vi "Traction Receipe Trial.vi"() -> ()   [LabVIEW 2025]
panel:
  out "sum":dbl
  in  "SRR Sweep Range (%) 2":string caption="Speed (mm/s)"
  in  "Multicolumn Listbox":i32(listbox)
  in  "Total Execution Time":dbl
  in  "Total Steps":dbl
  in  "Duration / Step (s)":dbl=6.0
  in  "STRIBECK Fixed SRR List (%)":string="5,10,20,40,60,80,100"
  in  "Duration / Step (s)":dbl=6.0
  in  "SRR Sweep Range (%)":string
  in  "Rolling Speed (mm/s)":dbl=1000.0
  in  "Temperature Stages (°C)":string="40,100,140"
  in  "Ball Load (N)":string="25"
  in  "Lubricant Name":string
  in  "Profile File Name":string
  # "1. Test Identification & Global Setup"
  # "2. Step Configurations & Timing"
  # "Step 1 Configuration: TRACTION Step"
  # "%"
  # "Steps 2+ Configuration: STRIBECK Steps"
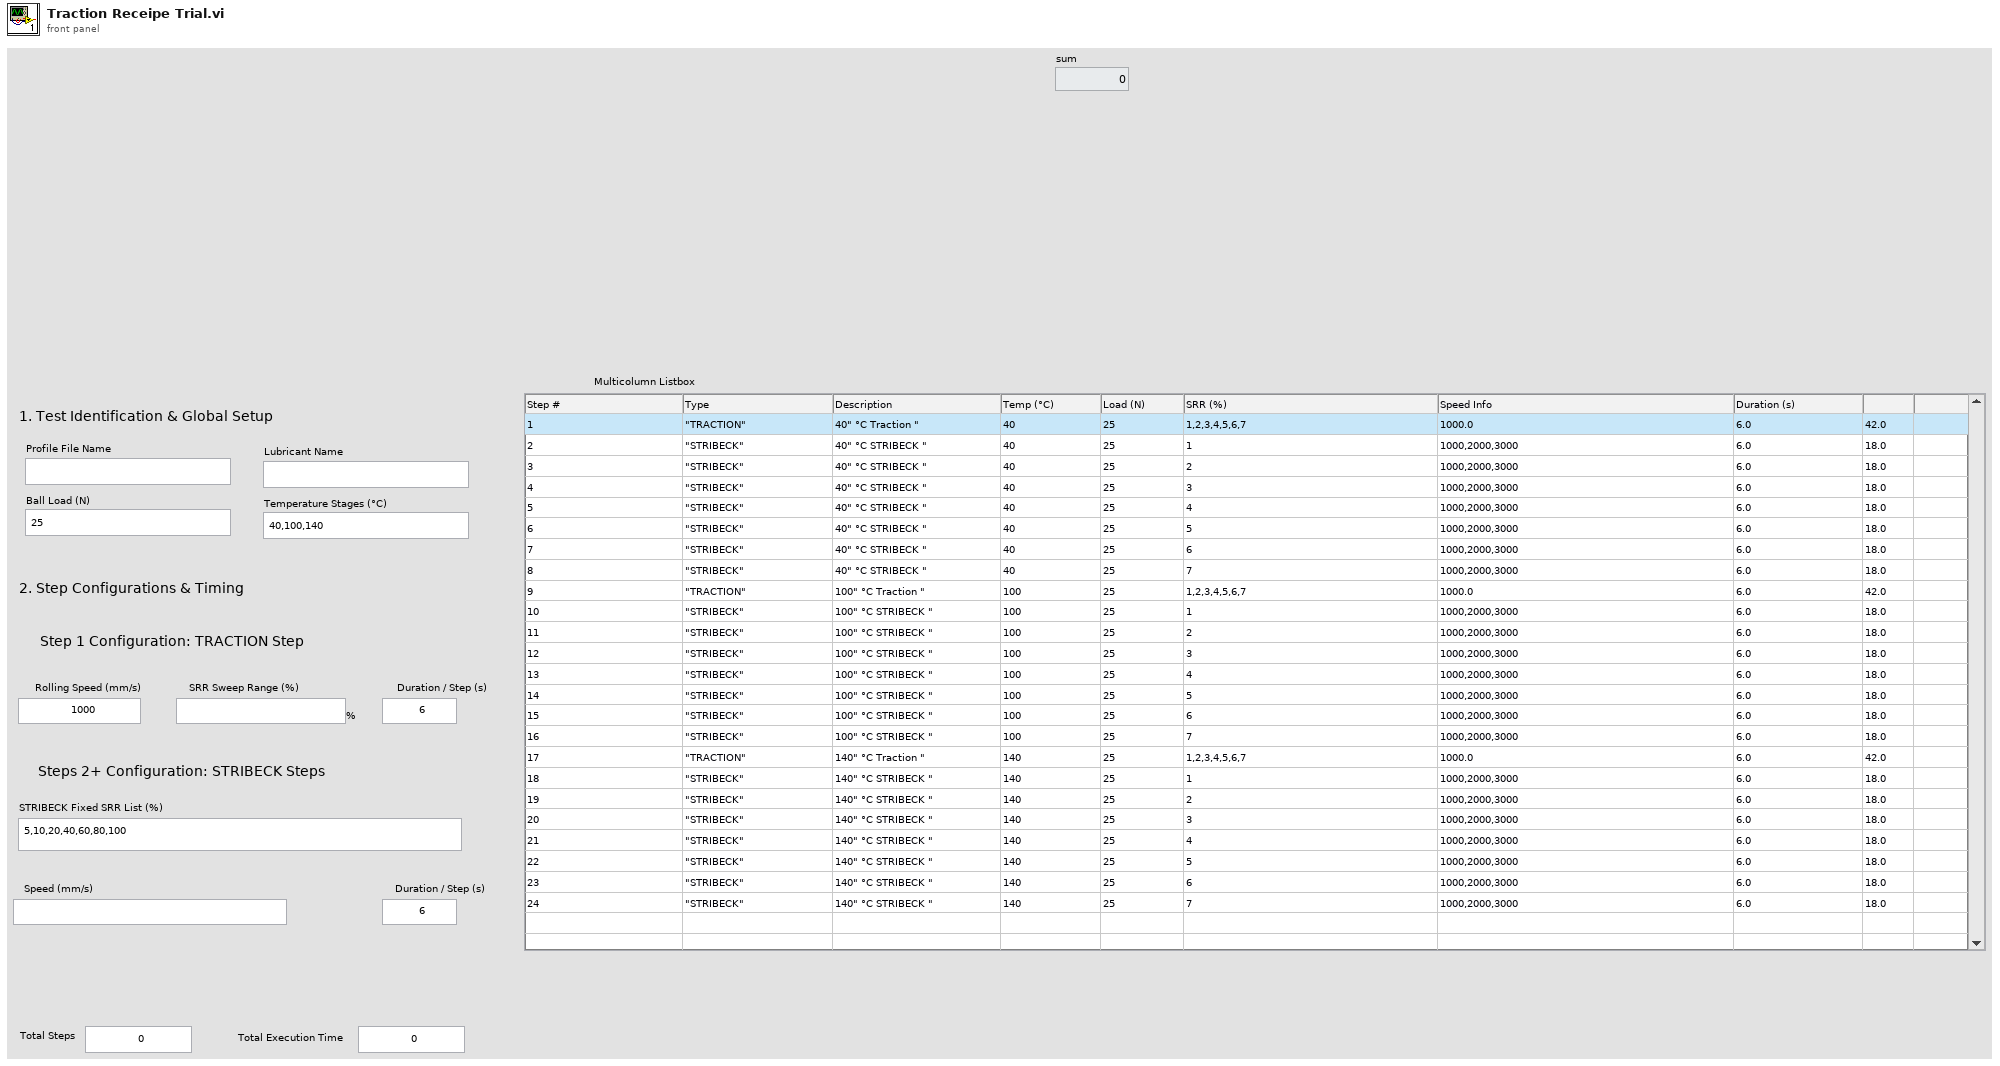
[diagram p1: front panel]
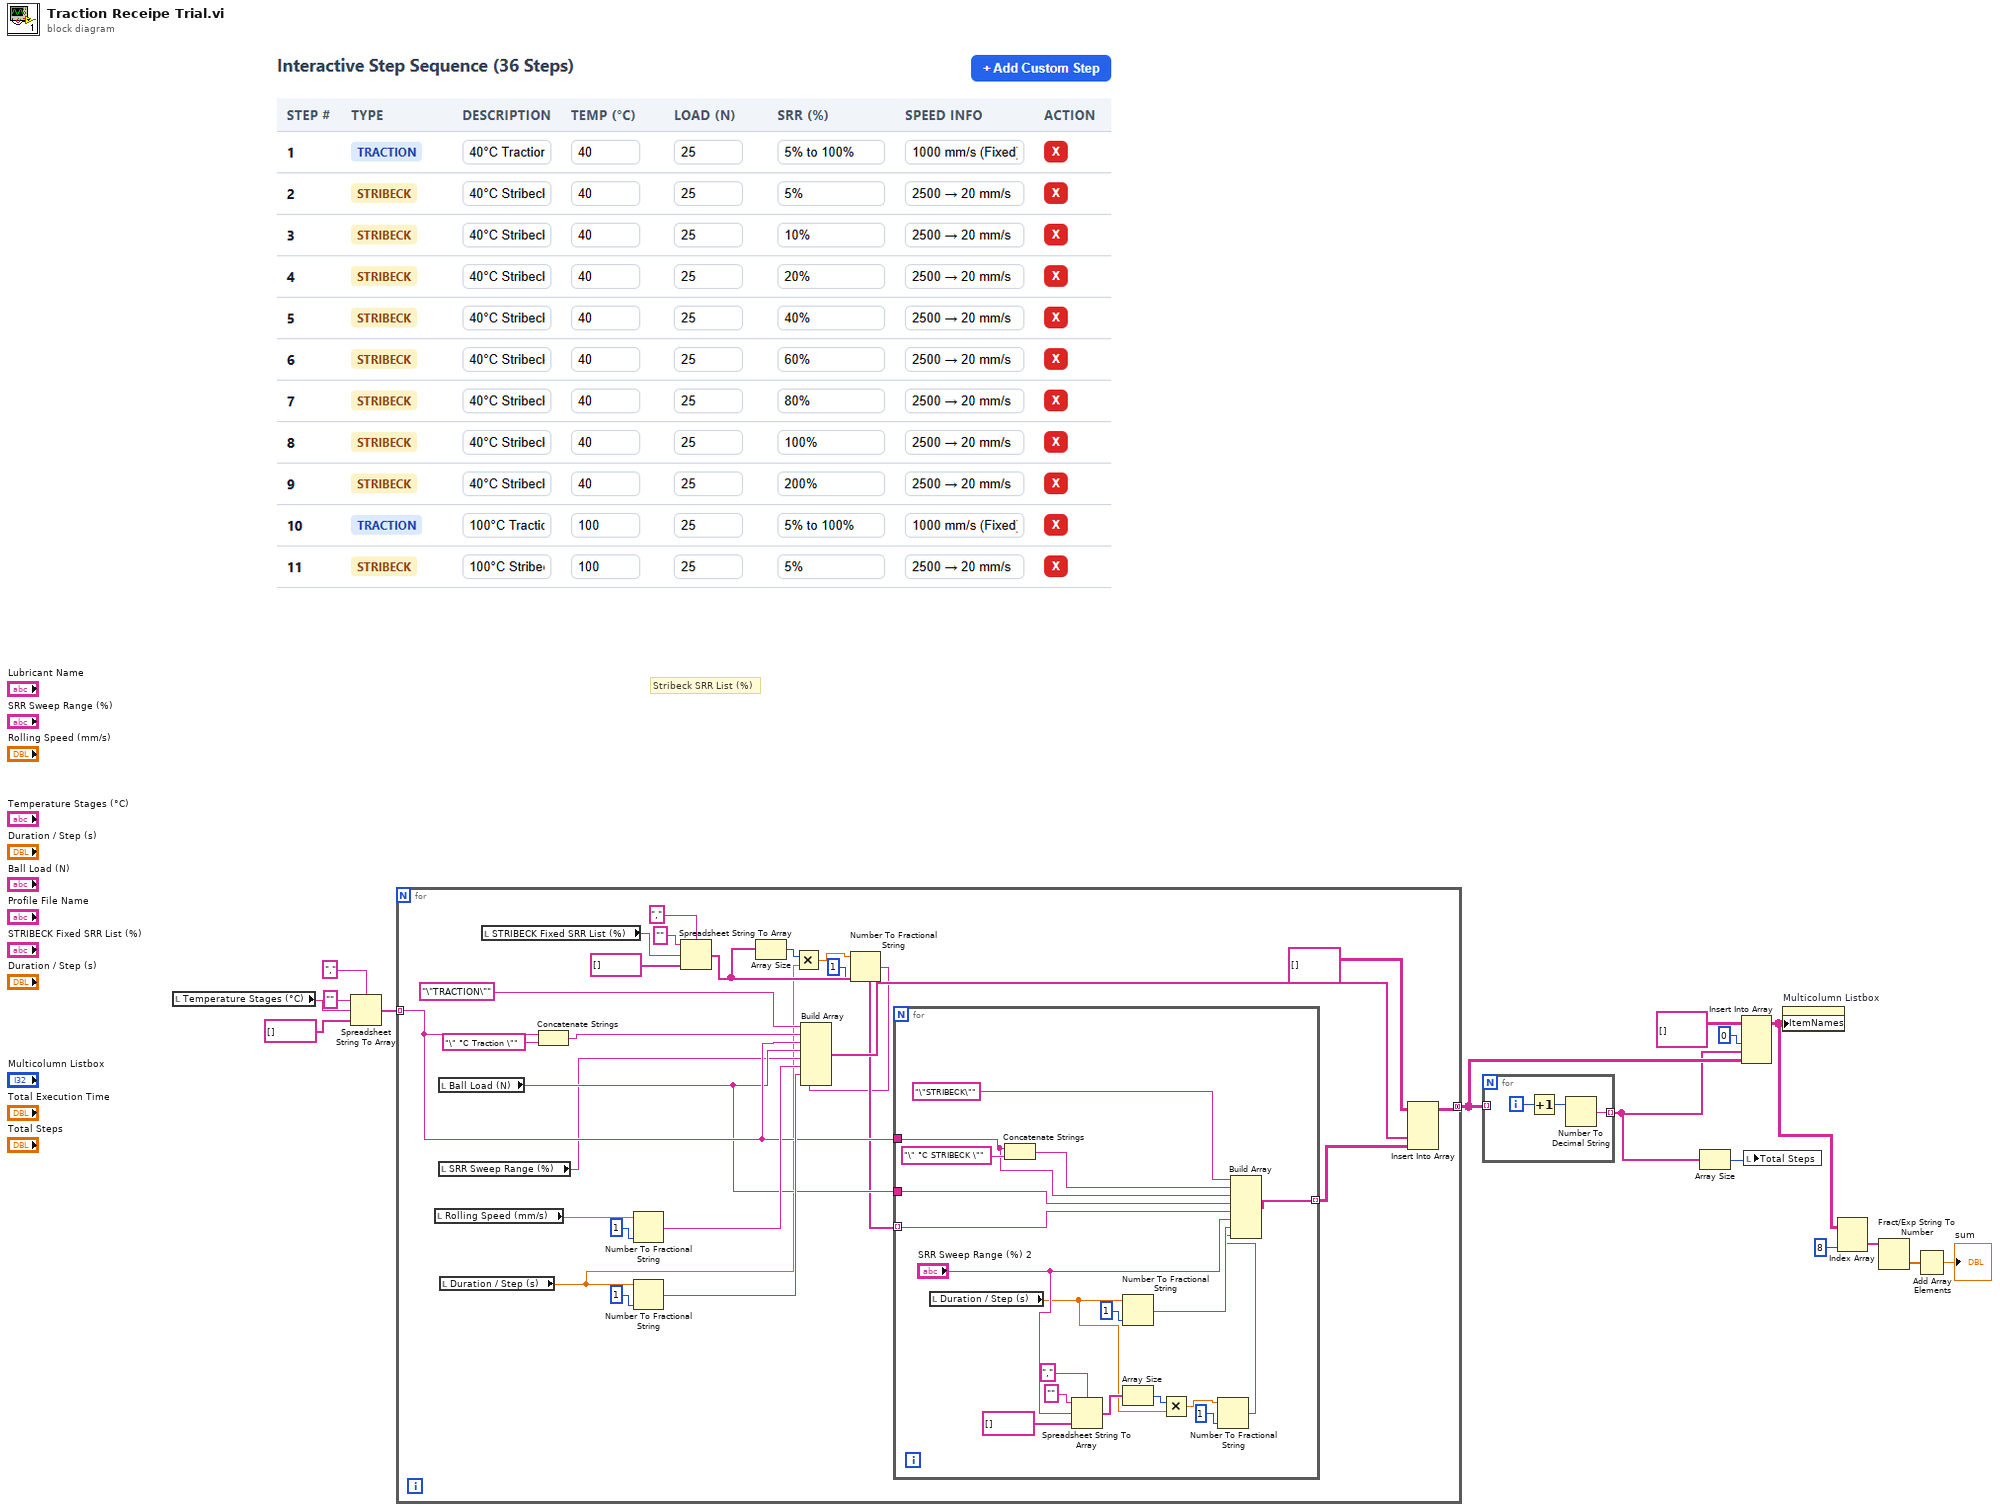
[diagram p0: block diagram]
diagram:
  # "Stribeck SRR List (%)"
  n1 = local read "Temperature Stages (°C)"() -> (w15:string)
  n2 = Spreadsheet String To Array(delimiter (Tab)=",", format string="", spreadsheet string=w15, array type (2D Dbl)=string[] []) -> (array=w11:string[])
  n3 = for {
    tunnel: w11 -> [w28] mode=indexing
    tunnel: [w23] -> w8 mode=concatenating
    n4 = local read "Rolling Speed (mm/s)"() -> (w38:dbl)
    n5 = local read "Ball Load (N)"() -> (w27:string)
    n6 = local read "SRR Sweep Range (%)"() -> (w22:string)
    n7 = local read "Duration / Step (s)"() -> (w19:dbl)
    n8 = local read "STRIBECK Fixed SRR List (%)"() -> (w32:string)
    n9 = Concatenate Strings(w28, "\" °C Traction \"" ("string")) -> (w35:string)
    n10 = Number To Fractional String(number=w38, precision (6)=i16 1) -> (F-format string=w34:string)  [unwired: 2 in]
    n11 = Number To Fractional String(number=w19, precision (6)=i16 1) -> (F-format string=w33:string)  [unwired: 2 in]
    n12 = Spreadsheet String To Array(delimiter (Tab)=",", format string="", spreadsheet string=w32, array type (2D Dbl)=string[] []) -> (array=w21:string[])
    n13 = Array Size(array=w21) -> (size(s)=w20:i32)
    n14 = Multiply(x=w20, y=w19) -> (x*y=w17:dbl)
    n15 = Number To Fractional String(number=w17, precision (6)=i16 1) -> (F-format string=w16:string)  [unwired: 2 in]
    n16 = Build Array("\"TRACTION\"", w35, w28, w27, w22, w34, w33, w16) -> (w25:string[])
    n17 = for {
      tunnel: w21 -> [w53] mode=indexing
      tunnel: w28 -> [w55]
      tunnel: w27 -> [w54]
      tunnel: [w51] -> w24 mode=indexing
      n18 = local read "Duration / Step (s)"() -> (w42:dbl)
      n19 = Concatenate Strings(w55, "\" °C STRIBECK \"" ("string")) -> (w56:string)
      n20 = Spreadsheet String To Array(delimiter (Tab)=",", format string="", spreadsheet string="SRR Sweep Range (%) 2", array type (2D Dbl)=string[] []) -> (array=w43:string[])
      n21 = Number To Fractional String(number=w42, precision (6)=i16 1) -> (F-format string=w52:string)  [unwired: 2 in]
      n22 = Array Size(array=w43) -> (size(s)=w46:i32)
      n23 = Multiply(x=w46, y=w42) -> (x*y=w44:dbl)
      n24 = Number To Fractional String(number=w44, precision (6)=i16 1) -> (F-format string=w41:string)  [unwired: 2 in]
      n25 = Build Array("\"STRIBECK\"", w56, w55, w54, w53, "SRR Sweep Range (%) 2", w52, w41) -> (w51:string[])
    }
    n26 = Insert Into Array(array=string[][] [] ("Array"), new element #1=w25, new element #2=w24) -> (w23:string[][])  [unwired: 2 in]
  }
  n27 = for {
    tunnel: w8 -> [_] mode=indexing
    tunnel: [w61] -> w7 mode=indexing
    i -> [w62]
    n28 = Increment(x=w62) -> (x+1=w60:i32)
    n29 = Number To Decimal String(number=w60) -> (decimal integer string=w61:string)  [unwired: 1 in]
  }
  n30 = Array Size(array=w7) -> (size(s)=w6:i32)
  n31 = Insert Into Array(array=string[][] [] ("Array"), index (col)=0 ("disabled index (col)"), new element #1=w7, new element #2=w8) -> (w4:string[][])  [unwired: 1 in]
  n32 = local write "Total Steps"(w6) -> ()
  n33 = property on="Multicolumn Listbox" class="MCListbox (strict)"("ItemNames"=w4) -> ()  [unwired: 2 in, 2 out]
  n34 = Index Array(array=w4, index (col)=8 ("disabled index (col)")) -> (element=w3:string[])  [unwired: 1 in]
  n35 = Fract/Exp String To Number(string=w3) -> (number=w2:dbl[])  [unwired: 3 in, 1 out]
  n36 = Add Array Elements(numeric array=w2) -> (sum=→"sum":dbl)
